vi "Threshold1DArraySafe.vi"(10 "HEIGHT":dbl, 11 "ampexp":dbl[](array[numeric])) -> (3 "Numeric":dbl)   [LabVIEW 2021]
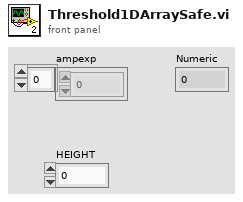
[diagram p1: front panel]
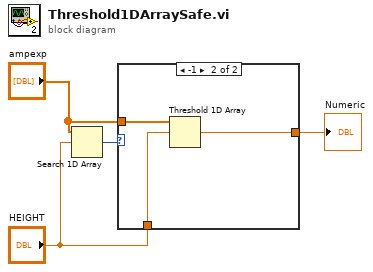
[diagram p0: block diagram]
diagram:
  n1 = Search 1D Array(1D array="ampexp", element="HEIGHT") -> (index of element=w1:i32)  [unwired: 1 in]
  n2 = case shown="-1" w1 {
    selector: w1 -> [w5 _]
    tunnel: [w5 w8] -> w4
    tunnel: "ampexp" -> [_ w7]
    tunnel: "HEIGHT" -> [_ w6]
    frame Default {
    }
    frame -1 {
      n3 = Threshold 1D Array(2:w6, 3:w7) -> (0:w8:dbl)  [unwired: 1 in]
    }
  }
  "Numeric" <- w4
